vi "Write Key (String).vi"(6 "Write Raw String? (F)":bool, 7 "Section Name":string, 8 "error in (no error)":errorcluster, 9 "Value":string, 10 "Key Name":string, 11 "Config in":refnum<class "LabVIEW-Config.lvclass">) -> (0 "error out":errorcluster, 2 "Key Replaced?":bool, 3 "Config out":refnum<class "LabVIEW-Config.lvclass">)   [LabVIEW 2017, in "LabVIEW-Config.lvlib" / "LabVIEW-Config.lvclass"]
uses:
  LabVIEW-Config.lvclass
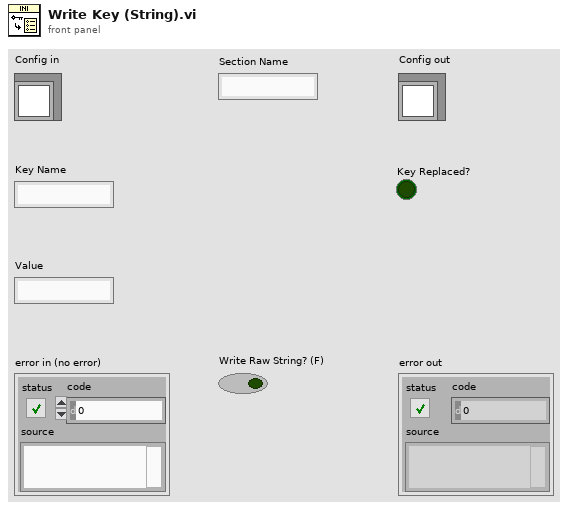
[diagram p1: front panel]
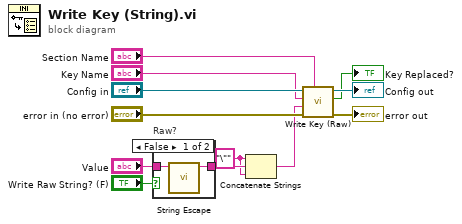
[diagram p0: block diagram]
diagram:
  w1 = "\"" ("string")
  n1 = case "Raw?" shown="False" "Write Raw String? (F)" {
    tunnel: "Value" -> [w14 w15]
    tunnel: [w13 w15] -> w3
    frame False {
      n2 = call "String Escape.vi"("Unescaped String"=w14) -> ("Escaped String"=w13:string)  [unwired: 10 in]
    }
    frame True {
    }
  }
  n3 = Concatenate Strings(w1, w3, w1) -> (w2:string)
  n4 = call "Write Key (Raw).vi"("Section Name"="Section Name", "error in (no error)"="error in (no error)", "Content"=w2, "Key Name"="Key Name", "Config in"="Config in") -> ("error out"=→"error out":errorcluster, "Key Replaced?"=→"Key Replaced?":bool, "Config out"=→"Config out":refnum<class "LabVIEW-Config.lvclass">)  [unwired: 4 in]
